vi "Waveplatecontrol.vi"() -> ()   [LabVIEW 2015]
uses:
  libs/Newport ESP301/Newport ESP301.lvlib
  <vilib>/DAQmx/write.llb/DAQmx Write (Analog DBL 1Chan 1Samp).vi
  <vilib>/DAQmx/create/channels.llb/DAQmx Create Channel (AO-Voltage-Basic).vi
panel:
  in  "ms2wait":u32
  in  "Boolean":bool
  out "a":waveform(dbl)(graph)={"t0"=timestamp(3634828212.0386066 s since 1904-01-01), "dt"=1.0, "Y"=[28.0]}
  out "Waveform Chart":dbl(graph)=5.25341140860948
  out "x*y":dbl=1.0
  in  "physical channels":tag="Dev3/ao1"
  out "DAC error":errorcluster
  out "ESP error":errorcluster
  out "run?":bool
  in  "set_vel":bool
  in  "velocity [fs/s]":dbl=66712.81903963041
  in  "vel_mm":dbl=10.0 caption="velocity [deg/s]"
  out "meas. velocity":dbl
  in  "stop":bool
  out "output voltage":dbl=1.0
  in  "start":bool
  in  "go2p1":bool
  out "position [deg]":dbl=28.0
  in  "p2 [deg]":dbl=2.0
  in  "p1 [deg]":dbl=28.0
  in  "interpolate output":bool
  in  "Delta2 [deg]":dbl=-173453.32950303904
  in  "Delta1 [deg]":dbl
  in  "Reference [deg]":dbl=28.0
  in  "Axis (1)":i32=2 min=1 max=3
  in  "Serial Link (RS232)":enum16{"RS232", "USB"}(ring)
  in  "VISA resource name":refnum<visa-resource-name>="COM9"
  in  "main_close":bool
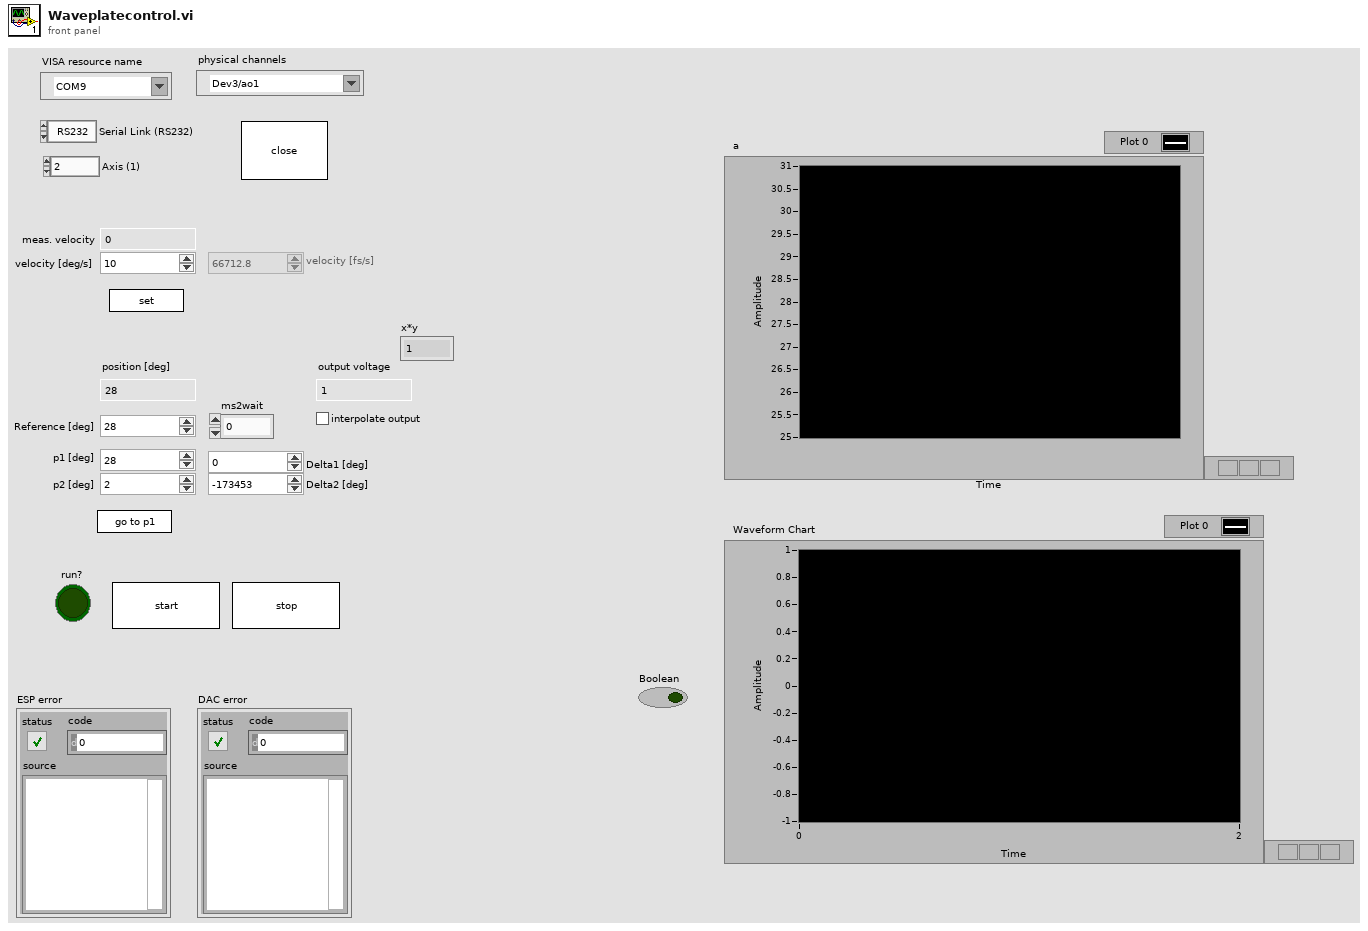
[diagram p1: front panel]
types:
  T1 = cluster{"dev1_data":refnum<queue>, "dev2_data":refnum<queue>}
  T2 = cluster{"dev1_cmd":refnum<queue>, "dev2_cmd":refnum<queue>}
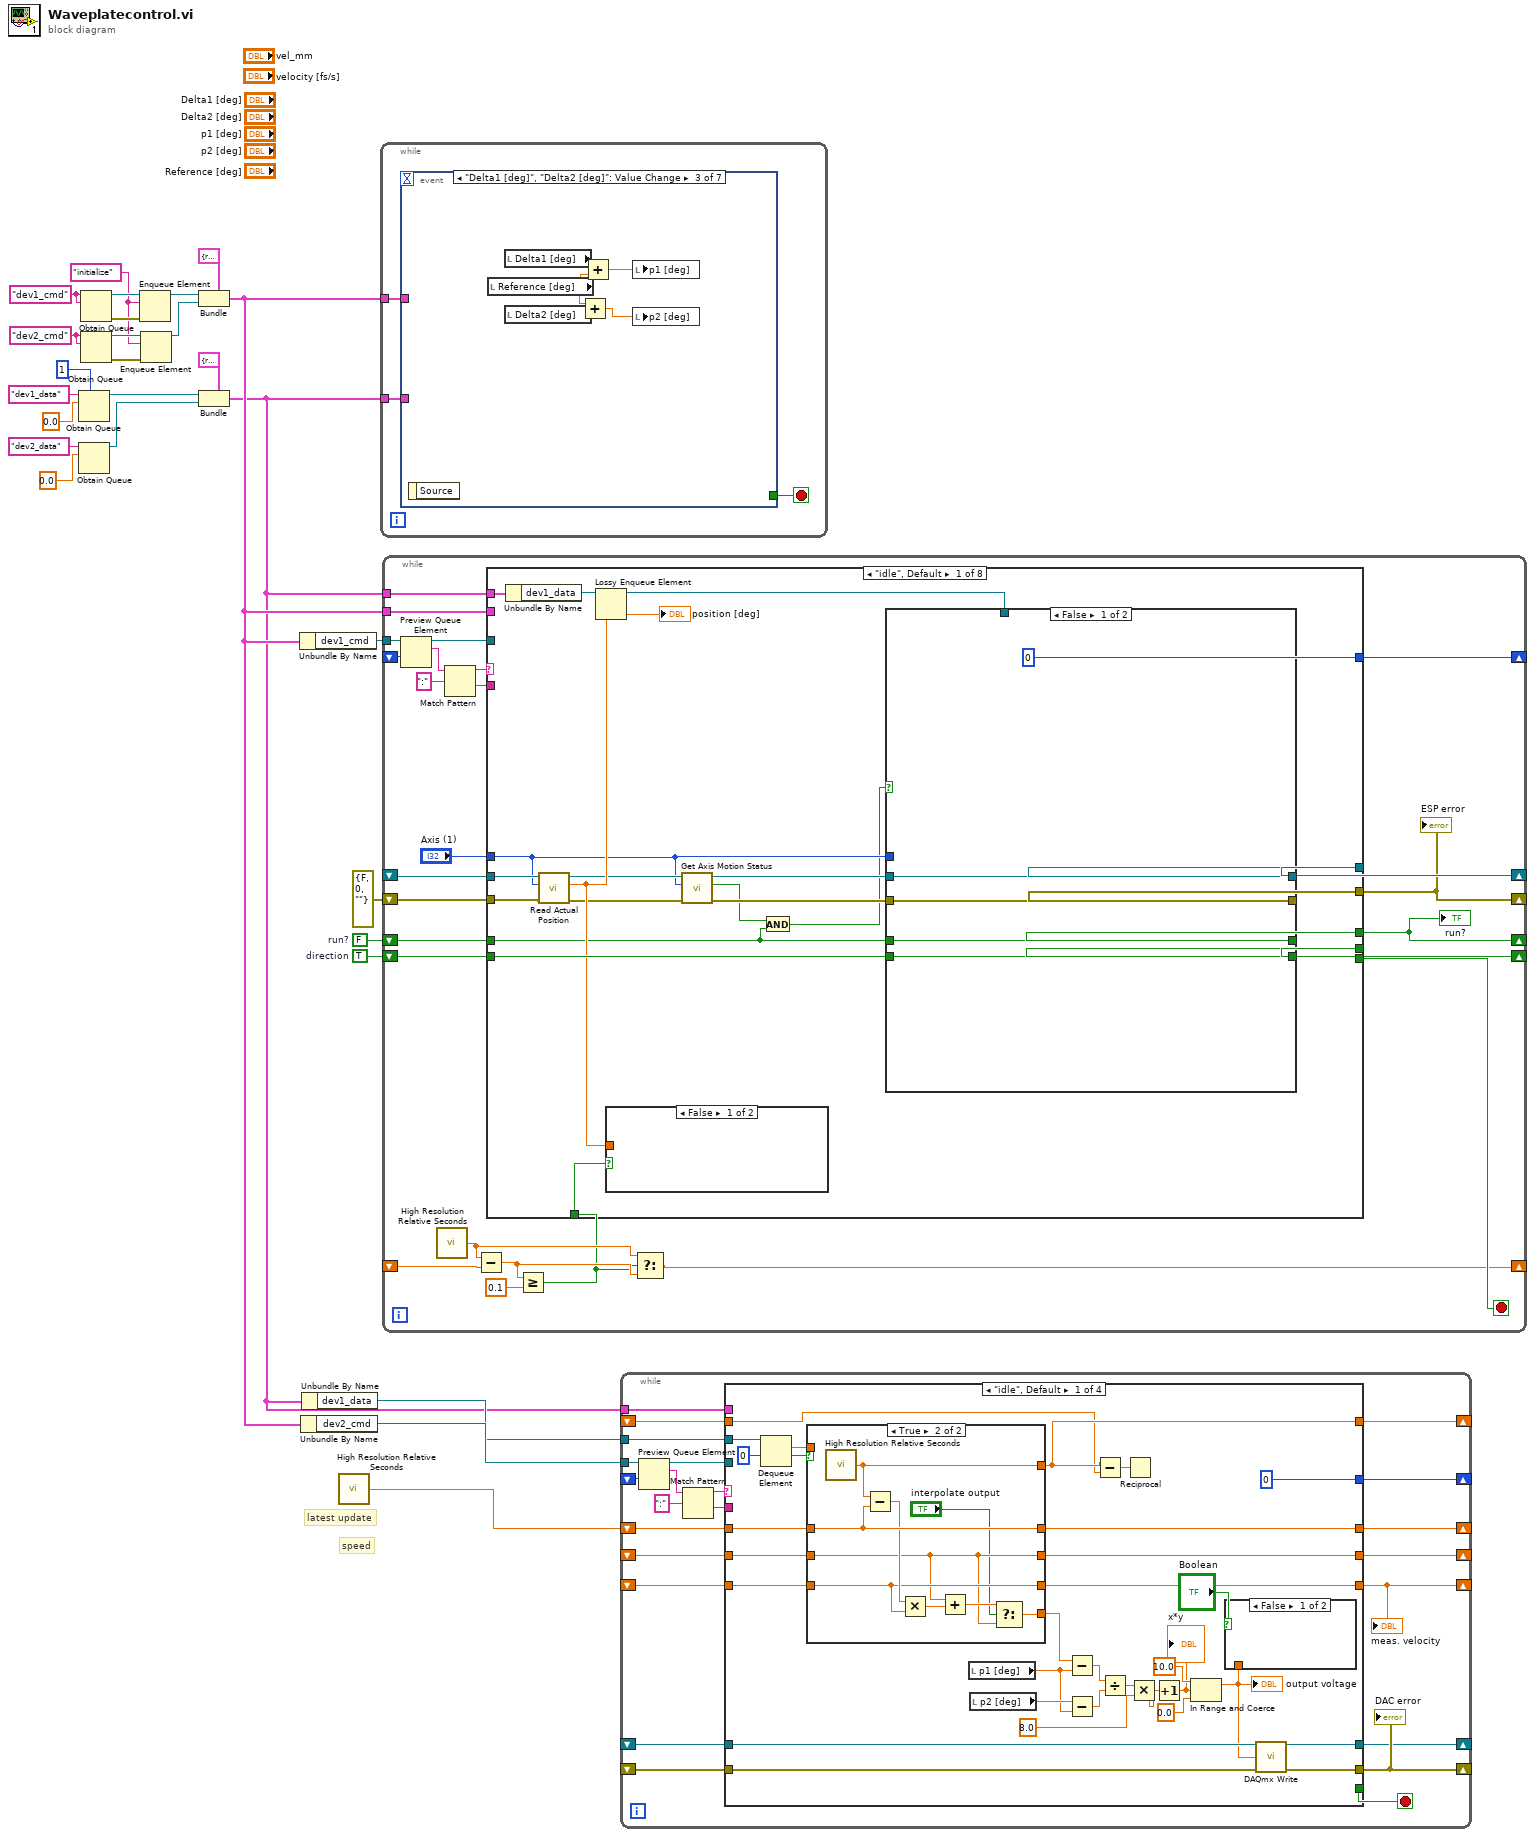
[diagram p0: block diagram]
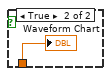
[diagram p2: hidden frame]
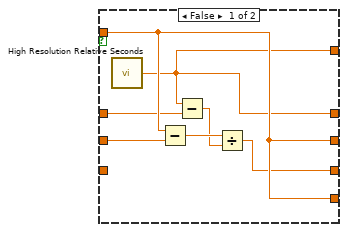
[diagram p3: hidden frame]
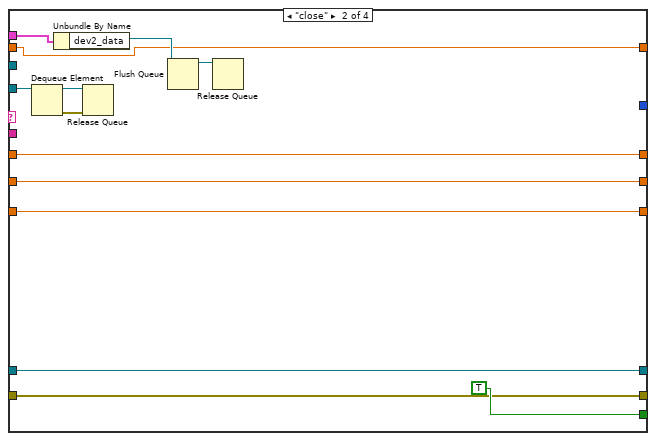
[diagram p4: hidden frame]
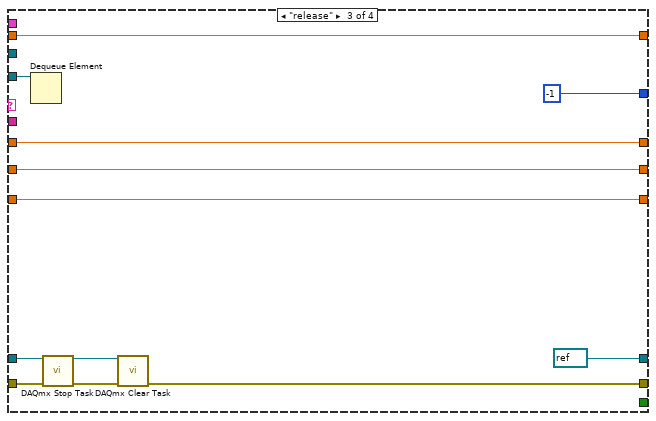
[diagram p5: hidden frame]
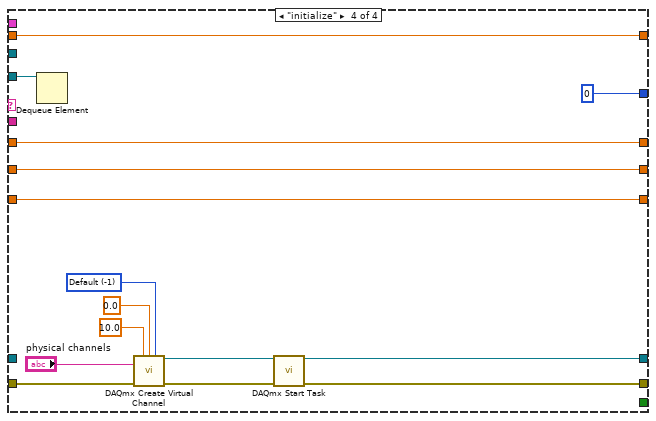
[diagram p6: hidden frame]
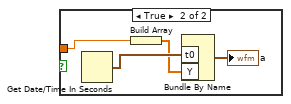
[diagram p7: hidden frame]
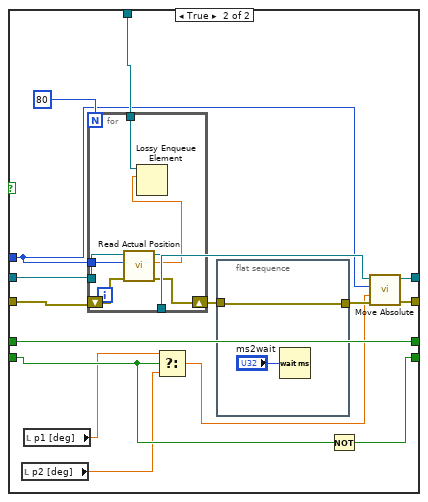
[diagram p8: hidden frame]
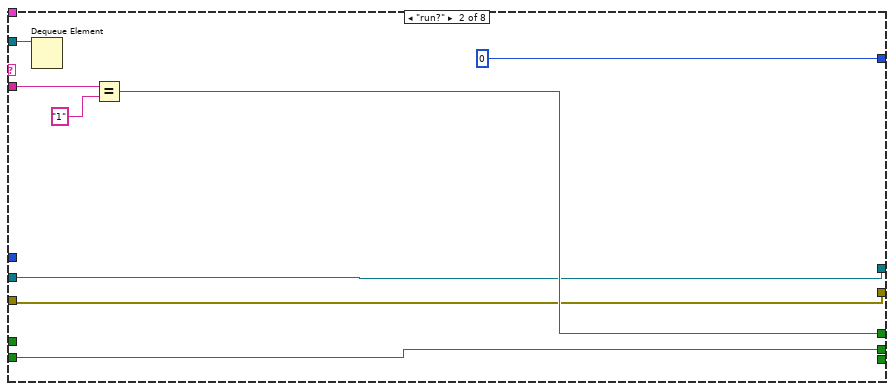
[diagram p9: hidden frame]
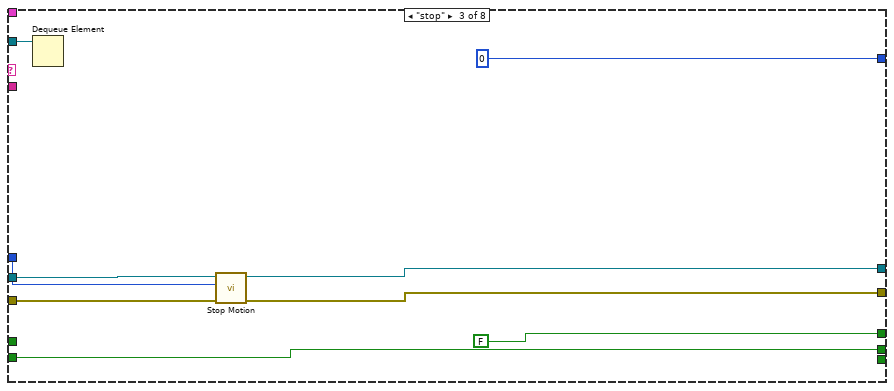
[diagram p10: hidden frame]
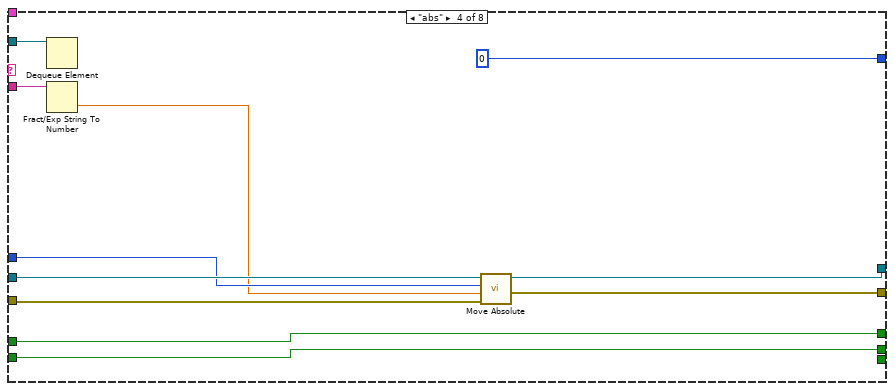
[diagram p11: hidden frame]
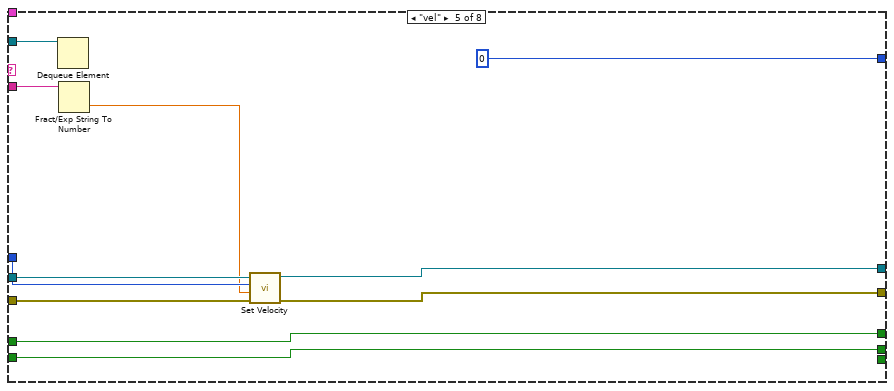
[diagram p12: hidden frame]
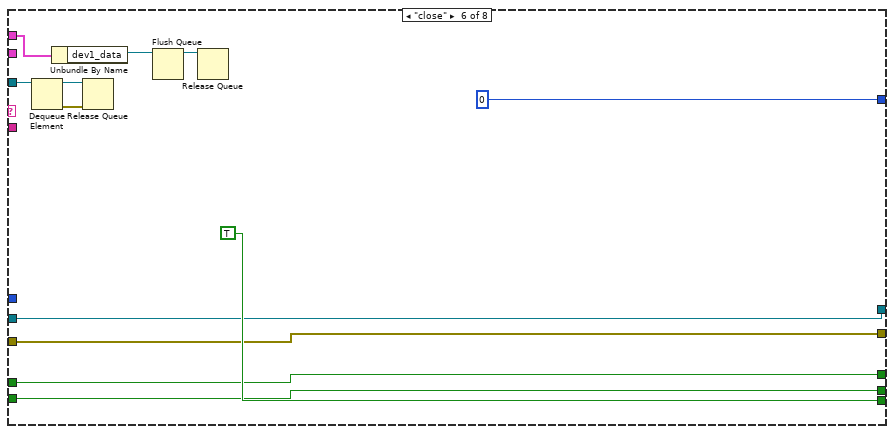
[diagram p13: hidden frame]
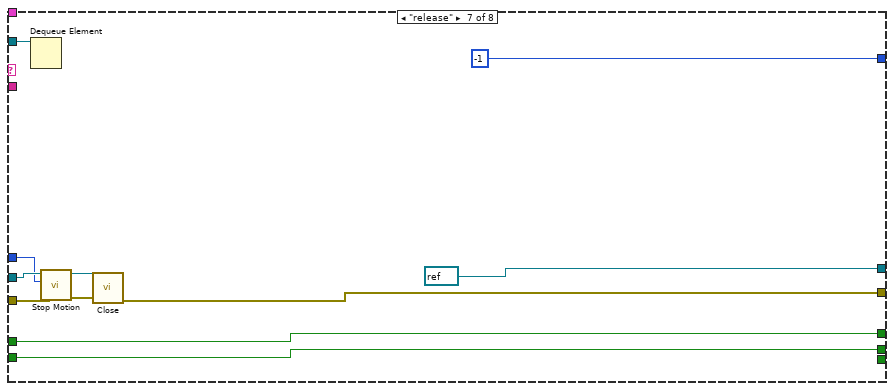
[diagram p14: hidden frame]
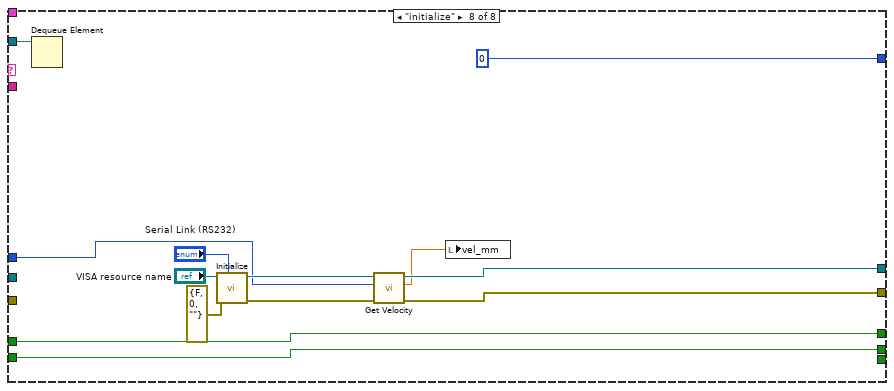
[diagram p15: hidden frame]
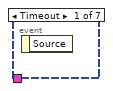
[diagram p16: hidden frame]
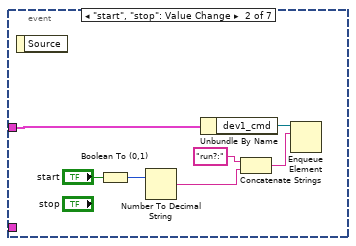
[diagram p17: hidden frame]
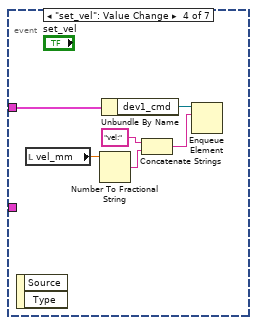
[diagram p18: hidden frame]
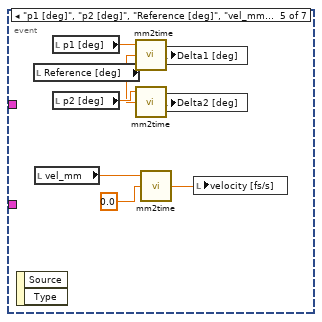
[diagram p19: hidden frame]
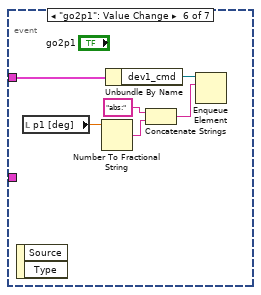
[diagram p20: hidden frame]
diagram:
  w1 = TRUE  # direction
  w4 = FALSE  # run?
  w15 = "dev2_cmd" ("name (unnamed)")
  w21 = "initialize" ("element")
  w16 = "dev1_cmd" ("name (unnamed)")
  # "speed"
  # "latest update"
  n1 = Obtain Queue(max queue size (-1, unlimited)=1, name (unnamed)="dev1_data", element data type=0.0) -> (queue out=w12:refnum<queue>)  [unwired: 2 in, 2 out]
  n2 = Obtain Queue(name (unnamed)="dev2_data", element data type=0.0) -> (queue out=w11:refnum<queue>)  [unwired: 3 in, 2 out]
  n3 = Obtain Queue(name (unnamed)=w16, element data type=w16) -> (queue out=w27:refnum<queue>, error out=w26:errorcluster)  [unwired: 3 in, 1 out]
  n4 = Obtain Queue(name (unnamed)=w15, element data type=w15) -> (queue out=w22:refnum<queue>, error out=w23:errorcluster)  [unwired: 3 in, 1 out]
  n5 = Enqueue Element(queue=w27, element=w21, error in (no error)=w26) -> (queue out=w24:refnum<queue>)  [unwired: 1 in, 2 out]
  n6 = Enqueue Element(queue=w22, element=w21, error in (no error)=w23) -> (queue out=w20:refnum<queue>)  [unwired: 1 in, 2 out]
  n7 = Bundle(cluster=T2 {"dev1_cmd"=refnum, "dev2_cmd"=refnum}, "dev1_cmd"=w24, "dev2_cmd"=w20) -> (w8:T2)
  n8 = Bundle(cluster=T1 {"dev1_data"=refnum, "dev2_data"=refnum}, "dev1_data"=w12, "dev2_data"=w11) -> (w2:T1)
  n9 = Unbundle By Name(w8) -> ("dev1_cmd"=w17:refnum<queue>)
  n10 = Unbundle By Name(w8) -> ("dev2_cmd"=w7:refnum<queue>)
  n11 = Unbundle By Name(w2) -> ("dev1_data"=w6:refnum<queue>)
  n12 = call <vilib>:"High Resolution Relative Seconds.vi"() -> ("relative seconds"=w5:dbl)
  n13 = while {
    tunnel: w8 -> [w30]
    tunnel: w2 -> [w29]
    stop <- w28 stop-if-true
    n14 = event shown="[2] \"Delta1 [deg]\", \"Delta2 [deg]\": Value Change" {
      selector: _ -> [_ _ _ _ _ _ _]
      dyn-events: _ -> [_ _ _ _ _ _ _]
      timeout: _ -> [_ _ _ _ _ _ _]
      tunnel: w30 -> [_ w34 _ w44 _ w62 w65]
      tunnel: w29 -> [_ _ _ _ _ _ _]
      tunnel: [_ _ _ _ _ _ TRUE] -> w28
      event Timeout {
        n15 = event-data() -> ()  [unwired: 1 in, 1 out]
      }
      event "start", "stop": Value Change {
        n16 = event-data() -> ()  [unwired: 1 in, 1 out]
        n17 = Boolean To (0,1)(Boolean="start") -> (0, 1=w32:i16)
        n18 = Number To Decimal String(number=w32) -> (decimal integer string=w31:string)  [unwired: 1 in]
        n19 = Unbundle By Name(w34) -> ("dev1_cmd"=w37:refnum<queue>)
        n20 = Concatenate Strings("run?:" ("string"), w31) -> (w36:string)
        n21 = Enqueue Element(queue=w37, element=w36) -> ()  [unwired: 2 in, 3 out]
      }
      event "Delta1 [deg]", "Delta2 [deg]": Value Change {
        n22 = event-data() -> ()  [unwired: 1 in, 1 out]
        n23 = local read "Reference [deg]"() -> (w40:dbl)
        n24 = local read "Delta1 [deg]"() -> (w42:dbl)
        n25 = local read "Delta2 [deg]"() -> (w41:dbl)
        n26 = Add(x=w40, y=w41) -> (x+y=w38:dbl)
        n27 = Add(x=w42, y=w40) -> (x+y=w39:dbl)
        n28 = local write "p1 [deg]"(w39) -> ()
        n29 = local write "p2 [deg]"(w38) -> ()
      }
      event "set_vel": Value Change {
        n30 = event-data() -> ()  [unwired: 1 in, 2 out]
        n31 = local read "vel_mm"() -> (w43:dbl)
        n32 = Number To Fractional String(number=w43) -> (F-format string=w47:string)  [unwired: 3 in]
        n33 = Unbundle By Name(w44) -> ("dev1_cmd"=w48:refnum<queue>)
        n34 = Concatenate Strings("vel:" ("string"), w47) -> (w46:string)
        n35 = Enqueue Element(queue=w48, element=w46) -> ()  [unwired: 2 in, 3 out]
      }
      event "p1 [deg]", "p2 [deg]", "Reference [deg]", "vel_mm": Value Change {
        n36 = event-data() -> ()  [unwired: 1 in, 2 out]
        n37 = local read "Reference [deg]"() -> (w54:dbl)
        n38 = local read "vel_mm"() -> (w51:dbl)
        n39 = local read "p1 [deg]"() -> (w55:dbl)
        n40 = local read "p2 [deg]"() -> (w56:dbl)
        n41 = call "mm2time.vi"("Offset (mm)"=w54, "distance (mm)"=w55) -> ("time in fs"=w52:dbl)  [unwired: 1 in]
        n42 = call "mm2time.vi"("Offset (mm)"=w54, "distance (mm)"=w56) -> ("time in fs"=w53:dbl)  [unwired: 1 in]
        n43 = call "mm2time.vi"("Offset (mm)"=0.0, "distance (mm)"=w51) -> ("time in fs"=w50:dbl)  [unwired: 1 in]
        n44 = local write "Delta1 [deg]"(w52) -> ()
        n45 = local write "Delta2 [deg]"(w53) -> ()
        n46 = local write "velocity [fs/s]"(w50) -> ()
      }
      event "go2p1": Value Change {
        n47 = event-data() -> ()  [unwired: 1 in, 2 out]
        n48 = local read "p1 [deg]"() -> (w57:dbl)
        n49 = Number To Fractional String(number=w57) -> (F-format string=w60:string)  [unwired: 3 in]
        n50 = Unbundle By Name(w62) -> ("dev1_cmd"=w61:refnum<queue>)
        n51 = Concatenate Strings("abs:" ("string"), w60) -> (w58:string)
        n52 = Enqueue Element(queue=w61, element=w58) -> ()  [unwired: 2 in, 3 out]
      }
      event "main_close": Value Change {
        n53 = event-data() -> ()  [unwired: 1 in, 1 out]
        n54 = Cluster To Array(cluster=w65) -> (array=w64:refnum<queue>[])
        n55 = for {
          tunnel: w64 -> [w70] mode=indexing
          n56 = Flush Queue(queue=w70) -> (queue out=w66:refnum<queue>)  [unwired: 1 in, 2 out]
          n57 = Enqueue Element(queue=w66, element="release") -> (queue out=w68:refnum<queue>)  [unwired: 2 in, 2 out]
          n58 = Enqueue Element(queue=w68, element="close") -> ()  [unwired: 2 in, 3 out]
        }
      }
    }
  }
  n59 = while {
    tunnel: w8 -> [w91]
    tunnel: w17 -> [w96]
    tunnel: w2 -> [w88]
    shift-right: [w86] -> _
    shift-left: _ -> [w87]
    shift-right: [w85] -> _
    shift-left: _ -> [w82]
    shift-right: [w84] -> _
    shift-left: errorcluster {"status"=FALSE, "code"=0, "source"=""} ("error out") -> [w83]
    shift-right: [w79] -> _
    shift-left: w4 -> [w80]
    shift-right: [w77] -> _
    shift-left: w1 -> [w78]
    shift-right: [w71] -> _
    shift-left: _ -> [w76]
    stop <- w89 stop-if-true
    n60 = Preview Queue Element(queue=w96, timeout in ms (-1)=w87) -> (queue out=w90:refnum<queue>, element=w95:string)  [unwired: 1 in, 2 out]
    n61 = call <vilib>:"High Resolution Relative Seconds.vi"() -> ("relative seconds"=w73:dbl)
    n62 = Match Pattern(string=w95, regular expression=":") -> (before substring=w93:string, after substring=w92:string)  [unwired: 1 in, 2 out]
    n63 = Subtract(x=w73, y=w76) -> (x-y=w74:dbl)
    n64 = Greater Or Equal?(x=w74, y=0.1) -> (x >= y?=w72:bool)
    n65 = case shown="\"idle\", Default" w93 {
      tunnel: w92 -> [_ w158 _ w177 w184 _ _ _]
      tunnel: w91 -> [_ _ _ _ _ _ _ _]
      tunnel: w90 -> [_ w156 w160 w178 w182 w201 w211 w221]
      tunnel: [_ _ _ _ _ TRUE _ _] -> w89
      tunnel: w88 -> [w116 _ _ _ _ w193 _ _]
      tunnel: [0 0 0 0 0 0 -1 0] -> w86
      tunnel: [w114 w151 w165 w174 w189 w197 refnum<visa-resource-name> refnum ("VISA resource name out") w217] -> w85
      tunnel: [w113 w152 w164 w173 w188 w196 w210 w216] -> w84
      tunnel: w83 -> [w111 w152 w166 w175 w187 w196 w206 _]
      tunnel: w82 -> [w112 w151 w167 w176 w186 w197 w203 _]
      tunnel: "Axis (1)" -> [w100 _ w163 w172 w185 _ w202 w218]
      tunnel: w80 -> [w98 _ _ w169 w180 w194 w208 w222]
      tunnel: [w108 w154 FALSE ("run?") w169 w180 w194 w208 w222] -> w79
      tunnel: w78 -> [w109 w153 w159 w168 w179 w190 w207 w213]
      tunnel: [w110 w153 w159 w168 w179 w190 w207 w213] -> w77
      tunnel: w72 -> [w107 _ _ _ _ _ _ _]
      frame "idle", Default {
        n66 = Unbundle By Name(w116) -> ("dev1_data"=w115:refnum<queue>)
        n67 = call "Read Actual Position.vi"("error in (no error)"=w111, "Axis (1)"=w100, "VISA resource name"=w112) -> ("error out"=w103:errorcluster, "Position (units)"=w105:dbl, "VISA resource name out"=w104:refnum<visa-resource-name>)  [unwired: 2 in]
        "position [deg]" <- w105
        n68 = Lossy Enqueue Element(queue=w115, element=w105) -> (queue out=w106:refnum<queue>)  [unwired: 1 in, 3 out]
        n69 = case shown="False" w107 {
          tunnel: w105 -> [_ w121]
          frame False {
          }
          frame True {
            n70 = Get Date/Time In Seconds() -> (seconds since 1Jan1904=w120:timestamp)
            n71 = Build Array(w121) -> (w119:dbl[])
            n72 = Bundle By Name("t0"=w120, "Y"=w119) -> (→"a":waveform(dbl))  [unwired: 1 in]
          }
        }
        n73 = call "Get Axis Motion Status.vi"("error in (no error)"=w103, "Axis (1)"=w100, "VISA resource name"=w104) -> ("error out"=w101:errorcluster, "Motion Done"=w99:bool, "VISA resource name out"=w102:refnum<visa-resource-name>)  [unwired: 2 in]
        n74 = And(x=w99, y=w98) -> (x .and. y?=w97:bool)
        n75 = case shown="False" w97 {
          tunnel: w102 -> [w125 w137]
          tunnel: w101 -> [w124 w138]
          tunnel: [w125 w135] -> w114
          tunnel: [w124 w134] -> w113
          tunnel: w100 -> [_ w131]
          tunnel: [w123 w129] -> w110
          tunnel: w109 -> [w123 w128]
          tunnel: w98 -> [w122 w141]
          tunnel: [w122 w141] -> w108
          tunnel: w106 -> [_ w140]
          frame False {
          }
          frame True {
            n76 = local read "p2 [deg]"() -> (w126:dbl)
            n77 = local read "p1 [deg]"() -> (w127:dbl)
            n78 = for {
              N: 80 -> [_]
              tunnel: w137 -> [w150]
              tunnel: [w149] -> w133
              shift-right: [w144] -> w136
              shift-left: w138 -> [w148]
              tunnel: w131 -> [w147]
              tunnel: w140 -> [w146]
              n79 = call "Read Actual Position.vi"("error in (no error)"=w148, "Axis (1)"=w147, "VISA resource name"=w150) -> ("error out"=w144:errorcluster, "Position (units)"=w145:dbl, "VISA resource name out"=w149:refnum<visa-resource-name>)  [unwired: 2 in]
              n80 = Lossy Enqueue Element(queue=w146, element=w145) -> ()  [unwired: 1 in, 4 out]
            }
            n81 = Select(t=w127, s=w128, f=w126) -> (s? t:f=w130:dbl)
            n82 = flat-sequence {
              tunnel: w136 -> [w143]
              tunnel: [w143] -> w132
              frame #0 {
                n83 = Wait (ms)(milliseconds to wait="ms2wait") -> ()  [unwired: 1 out]
              }
            }
            n84 = Not(x=w128) -> (.not. x?=w129:bool)
            n85 = call "Move Absolute.vi"("error in (no error)"=w132, "Position (0 units)"=w130, "Axis (1)"=w131, "VISA resource name"=w133) -> ("error out"=w134:errorcluster, "VISA resource name out"=w135:refnum<visa-resource-name>)  [unwired: 2 in]
          }
        }
      }
      frame "run?" {
        n86 = Dequeue Element(queue=w156) -> ()  [unwired: 2 in, 4 out]
        n87 = Equal?(x=w158, y="1") -> (x = y?=w154:bool)
      }
      frame "stop" {
        n88 = Dequeue Element(queue=w160) -> ()  [unwired: 2 in, 4 out]
        n89 = call "Stop Motion.vi"("error in (no error)"=w166, "Axis (1)"=w163, "VISA resource name"=w167) -> ("error out"=w164:errorcluster, "VISA resource name out"=w165:refnum<visa-resource-name>)  [unwired: 3 in]
      }
      frame "abs" {
        n90 = Dequeue Element(queue=w178) -> ()  [unwired: 2 in, 4 out]
        n91 = Fract/Exp String To Number(string=w177) -> (number=w171:dbl)  [unwired: 3 in, 1 out]
        n92 = call "Move Absolute.vi"("error in (no error)"=w175, "Position (0 units)"=w171, "Axis (1)"=w172, "VISA resource name"=w176) -> ("error out"=w173:errorcluster, "VISA resource name out"=w174:refnum<visa-resource-name>)  [unwired: 2 in]
      }
      frame "vel" {
        n93 = Dequeue Element(queue=w182) -> ()  [unwired: 2 in, 4 out]
        n94 = Fract/Exp String To Number(string=w184) -> (number=w183:dbl)  [unwired: 3 in, 1 out]
        n95 = call "Set Velocity.vi"("error in (no error)"=w187, "Velocity (units/s)"=w183, "Axis (1)"=w185, "VISA resource name"=w186) -> ("error out"=w188:errorcluster, "VISA resource name out"=w189:refnum<visa-resource-name>)  [unwired: 2 in]
      }
      frame "close" {
        n96 = Dequeue Element(queue=w201) -> (queue out=w200:refnum<queue>, error out=w199:errorcluster)  [unwired: 2 in, 2 out]
        n97 = Unbundle By Name(w193) -> ("dev1_data"=w191:refnum<queue>)
        n98 = Release Queue(queue=w200, error in (no error)=w199) -> ()  [unwired: 1 in, 3 out]
        n99 = Flush Queue(queue=w191) -> (queue out=w192:refnum<queue>)  [unwired: 1 in, 2 out]
        n100 = Release Queue(queue=w192) -> ()  [unwired: 2 in, 3 out]
      }
      frame "release" {
        n101 = Dequeue Element(queue=w211) -> ()  [unwired: 2 in, 4 out]
        n102 = call "Stop Motion.vi"("error in (no error)"=w206, "Axis (1)"=w202, "VISA resource name"=w203) -> ("error out"=w205:errorcluster, "VISA resource name out"=w204:refnum<visa-resource-name>)  [unwired: 3 in]
        n103 = call "Close.vi"("error in (no error)"=w205, "VISA resource name"=w204) -> ("error out"=w210:errorcluster)  [unwired: 9 in]
      }
      frame "initialize" {
        n104 = Dequeue Element(queue=w221) -> ()  [unwired: 2 in, 4 out]
        n105 = call "Initialize.vi"("VISA resource name"="VISA resource name", "error in (no error)"=errorcluster {"status"=FALSE, "code"=0, "source"=""}, "Serial Link (RS232)"="Serial Link (RS232)") -> ("VISA resource name out"=w220:refnum<visa-resource-name>, "error out"=w219:errorcluster)  [unwired: 6 in]
        n106 = call "Get Velocity.vi"("error in (no error)"=w219, "Axis (1)"=w218, "VISA resource name"=w220) -> ("error out"=w216:errorcluster, "Velocity (units/s)"=w215:dbl, "VISA resource name out"=w217:refnum<visa-resource-name>)  [unwired: 2 in]
        n107 = local write "vel_mm"(w215) -> ()
      }
    }
    "run?" <- w79
    "ESP error" <- w84
    n108 = Select(t=w73, s=w72, f=w74) -> (s? t:f=w71:dbl)
  }
  n109 = while {
    shift-right: [w241] -> _
    shift-left: _ -> [w242]
    shift-right: [w240] -> _
    shift-left: _ -> [w239]
    tunnel: w7 -> [w238]
    shift-right: [w237] -> _
    shift-left: _ -> [w236]
    tunnel: w6 -> [w235]
    shift-right: [w234] -> _
    shift-left: _ -> [w231]
    shift-right: [w233] -> _
    shift-left: w5 -> [w232]
    shift-right: [w226] -> _
    shift-left: _ -> [w230]
    tunnel: w2 -> [w229]
    shift-right: [w228] -> _
    shift-left: _ -> [w227]
    stop <- w243 stop-if-true
    n110 = Preview Queue Element(queue=w238, timeout in ms (-1)=w242) -> (queue out=w244:refnum<queue>, element=w248:string)  [unwired: 1 in, 2 out]
    n111 = Match Pattern(string=w248, regular expression=":") -> (before substring=w246:string, after substring=w245:string)  [unwired: 1 in, 2 out]
    n112 = case shown="\"idle\", Default" w246 {
      tunnel: w245 -> [_ _ _ _]
      tunnel: w244 -> [_ w309 w320 w328]
      tunnel: [_ TRUE _ _] -> w243
      tunnel: [0 _ -1 0] -> w241
      tunnel: [w275 w305 w319 w329] -> w240
      tunnel: w239 -> [w273 w305 w316 w336]
      tunnel: [w276 w304 refnum<k21> refnum ("task out") w330] -> w237
      tunnel: w236 -> [w274 w304 w317 _]
      tunnel: w235 -> [w277 _ _ _]
      tunnel: [w271 w302 w312 w325] -> w234
      tunnel: [w270 w303 w313 w326] -> w233
      tunnel: w232 -> [w268 w303 w313 w326]
      tunnel: w231 -> [w269 w302 w312 w325]
      tunnel: [w267 w301 w311 w324] -> w226
      tunnel: w230 -> [w266 w301 w311 w324]
      tunnel: w229 -> [_ w298 _ _]
      tunnel: [w255 w297 w310 w322] -> w228
      tunnel: w227 -> [w254 w297 w310 w322]
      frame "idle", Default {
        n113 = Dequeue Element(queue=w277, timeout in ms (-1)=0) -> (element=w272:dbl, timed out?=w256:bool)  [unwired: 1 in, 2 out]
        n114 = case shown="True" w256 {
          tunnel: w272 -> [w287 _]
          tunnel: [w287 w289] -> w265
          tunnel: [w287 w291] -> w271
          tunnel: [w281 w296] -> w270
          tunnel: w269 -> [w286 w291]
          tunnel: w268 -> [w285 w296]
          tunnel: [w282 w293] -> w267
          tunnel: w266 -> [_ w293]
          tunnel: [w281 w288] -> w255
          frame False {
            n115 = call <vilib>:"High Resolution Relative Seconds.vi"() -> ("relative seconds"=w281:dbl)
            n116 = Subtract(x=w287, y=w286) -> (x-y=w284:dbl)
            n117 = Subtract(x=w281, y=w285) -> (x-y=w283:dbl)
            n118 = Divide(x=w284, y=w283) -> (x/y=w282:dbl)
          }
          frame True {
            n119 = call <vilib>:"High Resolution Relative Seconds.vi"() -> ("relative seconds"=w288:dbl)
            n120 = Subtract(x=w288, y=w296) -> (x-y=w295:dbl)
            n121 = Multiply(x=w295, y=w293) -> (x*y=w294:dbl)
            n122 = Add(x=w291, y=w294) -> (x+y=w292:dbl)
            n123 = Select(t=w292, s="interpolate output", f=w291) -> (s? t:f=w289:dbl)
          }
        }
        n124 = local read "p1 [deg]"() -> (w263:dbl)
        n125 = local read "p2 [deg]"() -> (w264:dbl)
        n126 = Subtract(x=w265, y=w263) -> (x-y=w262:dbl)
        n127 = Subtract(x=w264, y=w263) -> (x-y=w261:dbl)
        n128 = Subtract(x=w255, y=w254) -> (x-y=w253:dbl)
        n129 = Divide(x=w262, y=w261) -> (x/y=w260:dbl)
        n130 = Reciprocal(x=w253) -> ()  [unwired: 1 out]
        n131 = Multiply(x=w260, y=8.0) -> (x*y=w251:dbl)
        n132 = Increment(x=w251) -> (x+1=w250:dbl)
        "x*y" <- w250
        n133 = In Range and Coerce(upper limit=10.0, x=w250, lower limit=0.0) -> (coerced(x)=w252:dbl)  [unwired: 1 out]
        "output voltage" <- w252
        n134 = case shown="False" "Boolean" {
          tunnel: w252 -> [_ w280]
          frame False {
          }
          frame True {
            "Waveform Chart" <- w280
          }
        }
        n135 = call-poly <vilib>:"DAQmx Write.vi"("task/channels in"=w274, "data"=w252, "error in"=w273) -> ("task out"=w276:refnum<k21>, "error out"=w275:errorcluster)  [unwired: 10 in, 1 out]
      }
      frame "close" {
        n136 = Dequeue Element(queue=w309) -> (queue out=w308:refnum<queue>, error out=w307:errorcluster)  [unwired: 2 in, 2 out]
        n137 = Unbundle By Name(w298) -> ("dev2_data"=w299:refnum<queue>)
        n138 = Release Queue(queue=w308, error in (no error)=w307) -> ()  [unwired: 1 in, 3 out]
        n139 = Flush Queue(queue=w299) -> (queue out=w300:refnum<queue>)  [unwired: 1 in, 2 out]
        n140 = Release Queue(queue=w300) -> ()  [unwired: 2 in, 3 out]
      }
      frame "release" {
        n141 = Dequeue Element(queue=w320) -> ()  [unwired: 2 in, 4 out]
        n142 = call <vilib>:"DAQmx Stop Task.vi"("task/channels in"=w317, "error in"=w316) -> ("task out"=w315:refnum<k21>, "error out"=w314:errorcluster)  [unwired: 12 in]
        n143 = call <vilib>:"DAQmx Clear Task.vi"("task in"=w315, "error in"=w314) -> ("error out"=w319:errorcluster)  [unwired: 13 in]
      }
      frame "initialize" {
        w333 = -1 items=["Default"=-1, "RSE"=10083, "Differential"=10106, "Pseudodifferential"=12529] ("output terminal configuration")
        n144 = Dequeue Element(queue=w328) -> ()  [unwired: 2 in, 4 out]
        n145 = call-poly <vilib>:"DAQmx Create Virtual Channel.vi"("maximum value"=10.0, "minimum value"=0.0, "output terminal configuration"=w333, "physical channels"="physical channels", "error in"=w336) -> ("task out"=w332:refnum<k21>, "error out"=w331:errorcluster)  [unwired: 9 in]
        n146 = call <vilib>:"DAQmx Start Task.vi"("task/channels in"=w332, "error in"=w331) -> ("task out"=w330:refnum<k21>, "error out"=w329:errorcluster)  [unwired: 12 in]
      }
    }
    "meas. velocity" <- w226
    "DAC error" <- w240
  }
